vi "DAQ_PS Configure and Measure.vi"(0 "DAQmx Task In":refnum<k21>, 2 "Execution Settings":T4, 5 "Channel Settings":T7={"Voltage Setpoint(V)"=1.0, "Current Setpoint(A)"=0.1, "Remote Sense"=16095, "Idle Output Behavior"=15503, "Enable Output?"=TRUE} {"Idle Output Behavior" items=["Disable output when Task stopped"=15503, "Maintain Existing Value"=12528]; "Remote Sense" items=["Local"=16095, "Remote"=16096]; "Voltage Setpoint(V)" format="%.2p"; "Current Setpoint(A)" format="%.2p"}, 7 "Timing and Trigger Settings":T1={"Timing Settings"={"Sample Clock Source"="OnboardClock", "Sample Rate (Hz)"=10000.0, "Number of Samples"=1000, "Sample Timing Engine"=enum."Auto"}, "Trigger Settings"={"Trigger Select"=enum."No Trigger", "Digital Start Trigger Source"="", "Digital Start Trigger Edge"=10280}} {"Timing Settings"."Sample Rate (Hz)" format="%.2p"; "Trigger Settings"."Digital Start Trigger Edge" items=["Rising"=10280, "Falling"=10171]}, 11 "error in":errorcluster) -> (4 "DAQmx Task Out":refnum<k21>, 6 "Voltage Waveforms":waveform(dbl)(graph), 8 "Current Waveforms":waveform(dbl)(graph), 10 "Power Measurements":T6 {"Average Power (W)" format="%.2p"; "Max Power(W)" format="%.2p"; "Max Current Level(A)" format="%.2p"; "Max Voltage Level(V)" format="%.2p"}, 14 "Acquisition Time (s)":dbl format="%.2p", 15 "error out":errorcluster)   [LabVIEW 2021, in "DAQ_Power Supply Source and Measure.lvlib"]
doc: "Configures, Initiate and fetch results for power supply measurements"
uses:
  DAQ_Power Supply Source and Measure.lvlib
  Typedefs/Channel Settings.ctl
  Typedefs/Power Measurements.ctl
  Typedefs/Timing and Trigger Settings.ctl
  Typedefs/Timing Settings.ctl
  Typedefs/Trigger Settings.ctl
  Typedefs/Execution Settings.ctl
  Common/Typedefs/Execution Options - Measure.ctl
  <vilib>/DAQmx/read.llb/DAQmx Read (Power Wfm 1Chan NSamp).vi
  <vilib>/DAQmx/configure/timing.llb/DAQmx Timing (Sample Clock).vi
  <vilib>/DAQmx/configure/trigger.llb/DAQmx Start Trigger (Digital Edge).vi
  <vilib>/DAQmx/miscellaneous.llb/DAQmx Fill In Error Info.vi
  <resource>/objmgr/daqmx.rc
panel:
  # "Inputs"
  # "Outputs"
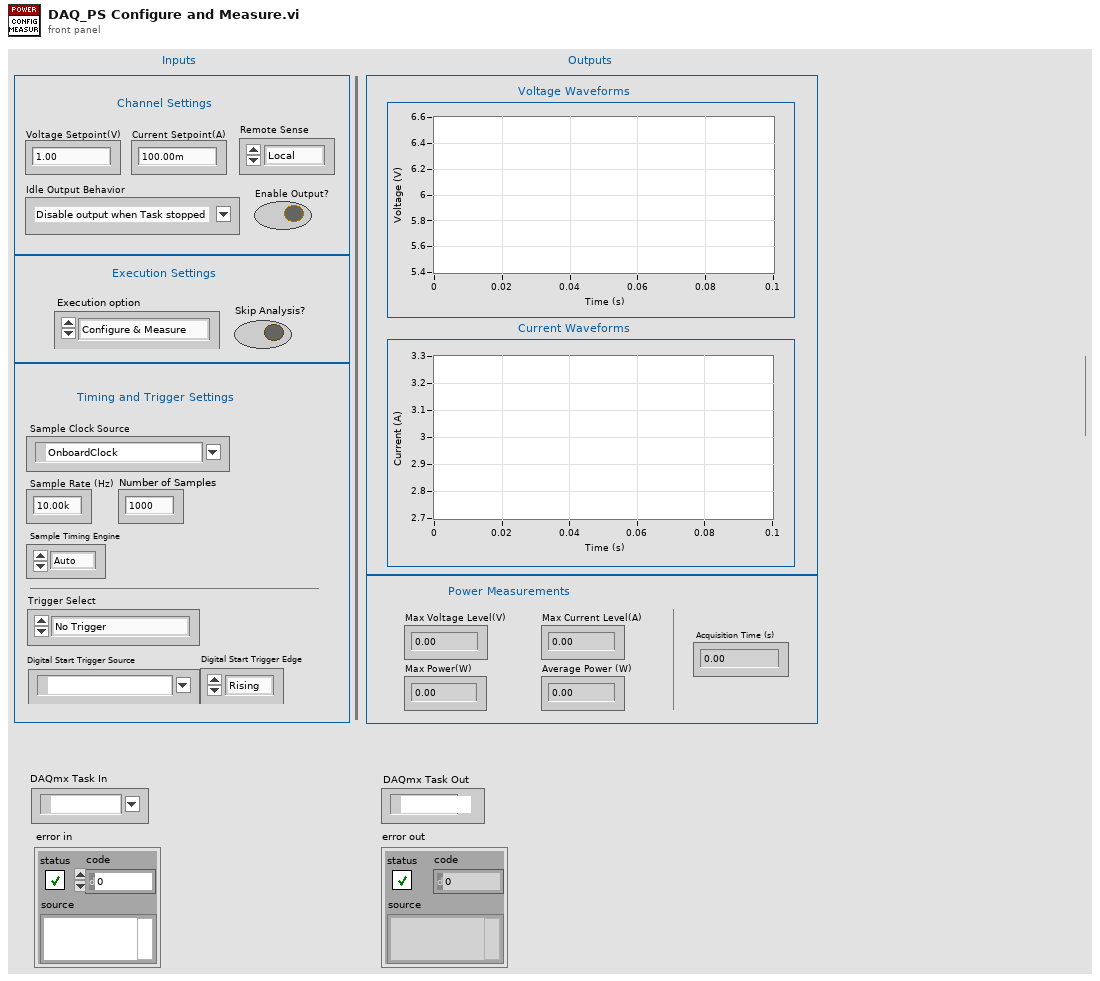
[diagram p1: front panel]
types:
  T1 = typedef "DAQ_Power Supply Source and Measure.lvlib/Timing and Trigger Settings.ctl" = cluster{"Timing Settings":T2, "Trigger Settings":T3}
  T2 = typedef "DAQ_Power Supply Source and Measure.lvlib/Timing Settings.ctl" = cluster{"Sample Clock Source":tag, "Sample Rate (Hz)":dbl, "Number of Samples":i32, "Sample Timing Engine":enum16{"te0", "te1", "ai", "Auto"}}
  T3 = typedef "DAQ_Power Supply Source and Measure.lvlib/Trigger Settings.ctl" = cluster{"Trigger Select":enum16{"No Trigger", "Digital Start"}, "Digital Start Trigger Source":tag, "Digital Start Trigger Edge":i32}
  T4 = typedef "DAQ_Power Supply Source and Measure.lvlib/Execution Settings.ctl" = cluster{"Execution option":T5, "Skip Analysis?":bool}
  T5 = typedef "Execution Options - Measure.ctl" = enum16{"Configure & Measure", "Configure only", "Measure only"}
  T6 = typedef "DAQ_Power Supply Source and Measure.lvlib/Power Measurements.ctl" = cluster{"Max Voltage Level(V)":dbl, "Max Current Level(A)":dbl, "Max Power(W)":dbl, "Average Power (W)":dbl}
  T7 = typedef "DAQ_Power Supply Source and Measure.lvlib/Channel Settings.ctl" = cluster{"Voltage Setpoint(V)":dbl, "Current Setpoint(A)":dbl, "Remote Sense":i32, "Idle Output Behavior":i32, "Enable Output?":bool}
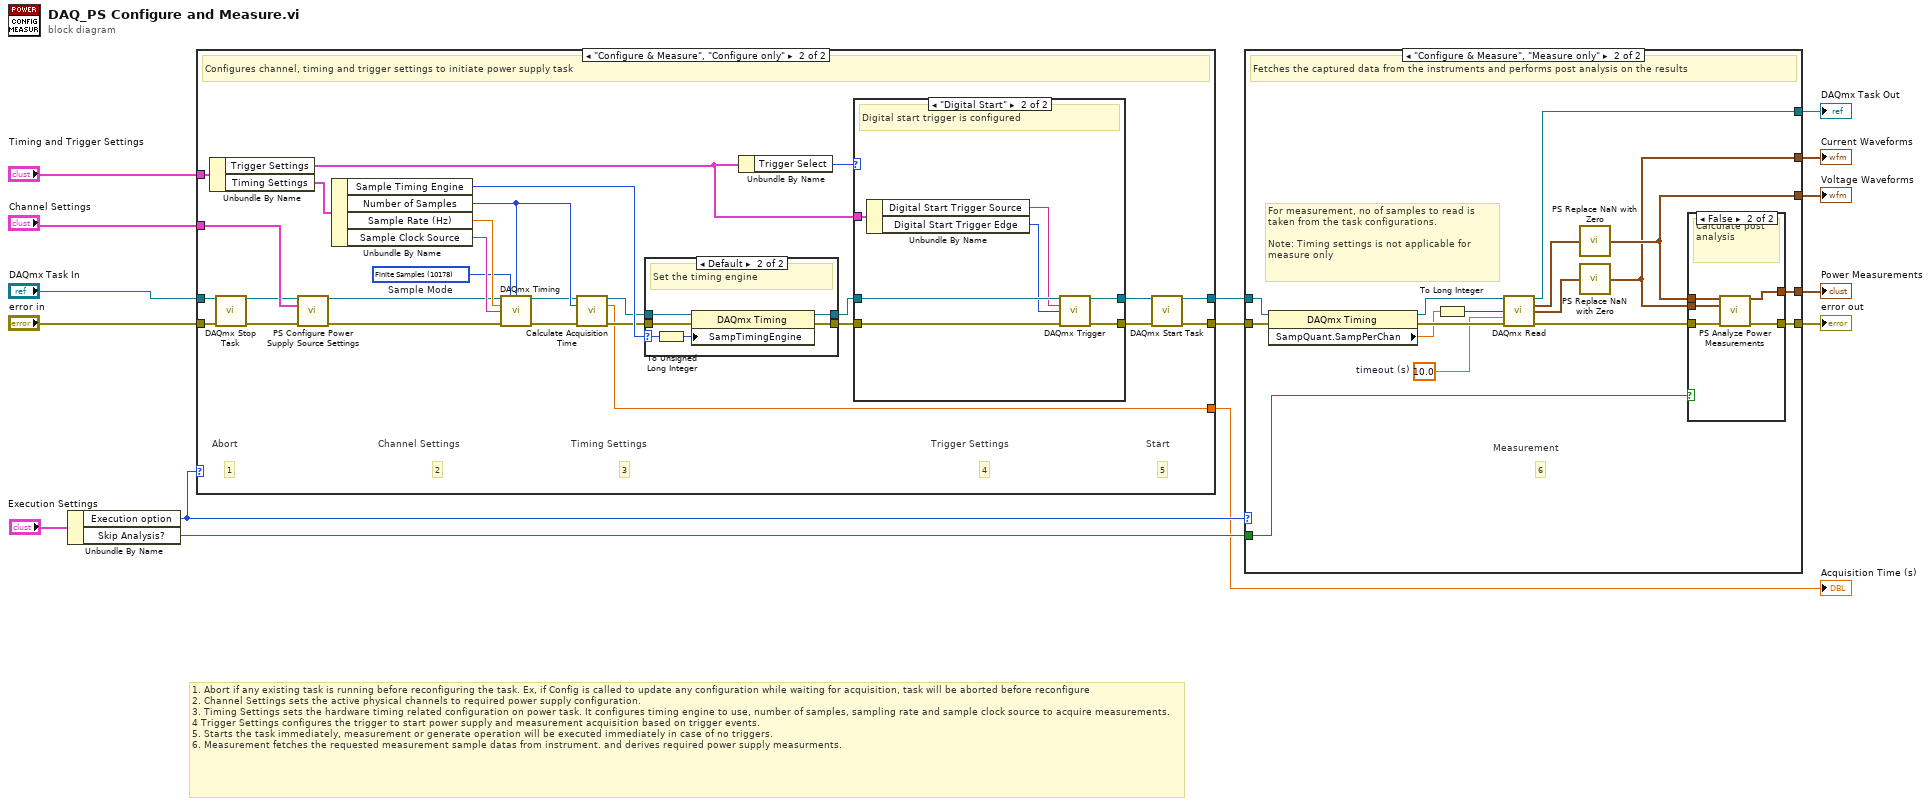
[diagram p0: block diagram]
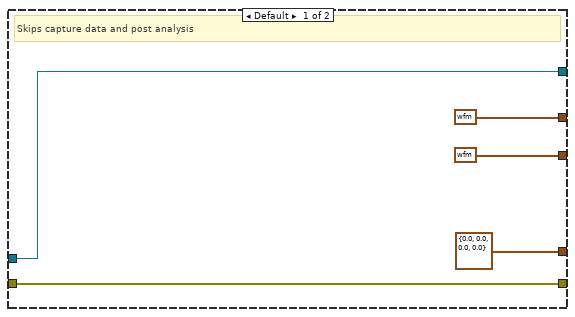
[diagram p5: hidden frame]
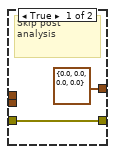
[diagram p6: hidden frame]
diagram:
  # "1. Abort if any existing task is running before reconfiguring the task. Ex, if Config is called to update any configuration while waiting for acquisition, task will be aborted before reconfigure\n2. Channel Settings sets the active physical channels to required power supply configuration.\n3. Timing Settings sets the hardware timing related configuration on power task. It configures timing engine to use, number of samples, sampling rate and sample clock source to acquire measurements.\n4 Trigger Settings configures the trigger to start power supply and measurement acquisition based on trigger events.\n5. Starts the task immediately, measurement or generate operation will be executed immediately in case of no triggers.\n6. Measurement fetches the requested measurement sample datas from instrument. and derives required power supply measurments."
  n1 = Unbundle By Name("Execution Settings") -> ("Execution option"=w5:T5, "Skip Analysis?"=w4:bool)
  n2 = case shown="\"Configure & Measure\", \"Configure only\"" w5 {
    tunnel: "Channel Settings" -> [_ w43]
    tunnel: "DAQmx Task In" -> [w16 w41]
    tunnel: "error in" -> [w17 w44]
    tunnel: [w16 w38] -> w10
    tunnel: [w17 w39] -> w9
    tunnel: "Timing and Trigger Settings" -> [_ w27]
    tunnel: [_ w18] -> w3
    frame Default {
      # "Configuration is skipped"
    }
    frame "Configure & Measure", "Configure only" {
      w29 = 10178 items=["Finite Samples"=10178, "Continuous Samples"=10123, "Hardware Timed Single Point"=12522]  # Sample Mode
      # "5"
      # "Start"
      # "1"
      # "Abort"
      # "4"
      # "Timing Settings"
      # "3"
      # "2"
      # "Trigger Settings"
      # "Channel Settings"
      # "Configures channel, timing and trigger settings to initiate power supply task"
      n3 = Unbundle By Name(w27) -> ("Trigger Settings"=w37:T3, "Timing Settings"=w35:T2)
      n4 = call <vilib>:"DAQmx Stop Task.vi"("task/channels in"=w41, "error in"=w44) -> ("task out"=w40:refnum<k21>, "error out"=w42:errorcluster)  [unwired: 12 in]
      n5 = call "PS Configure Power Supply Source Settings.vi"("DAQmx Task In"=w40, "Channel Settings"=w43, "error in (no error)"=w42) -> ("DAQmx Task Out"=w26:refnum<k21>, "error out"=w25:errorcluster)  [unwired: 11 in]
      n6 = Unbundle By Name(w35) -> ("Sample Timing Engine"=w34:enum16{"te0", "te1", "ai", "Auto"}, "Number of Samples"=w28:i32, "Sample Rate (Hz)"=w30:dbl, "Sample Clock Source"=w31:tag)
      n7 = call-poly <vilib>:"DAQmx Timing.vi"("task/channels in"=w26, "sample mode"=w29, "samples per channel"=w28, "rate"=w30, "source"=w31, "error in"=w25) -> ("task out"=w23:refnum<k21>, "error out"=w24:errorcluster)  [unwired: 8 in]
      n8 = call "Calculate Acquisition Time.vi"("Refnum in"=w23, "Number of Samples"=w28, "error in (no error)"=w24) -> ("Refnum out"=w21:refnum<k21>, "Acquisition Time Period (s)"=w18:dbl, "error out"=w22:errorcluster)  [unwired: 10 in]
      n9 = case shown="Default" w34 {
        selector: w34 -> [_ w50]
        tunnel: w22 -> [w46 w52]
        tunnel: w21 -> [w45 w51]
        tunnel: [w45 w49] -> w32
        tunnel: [w46 w48] -> w33
        frame "Auto" {
          # "Timing engine is auto-selected"
        }
        frame Default {
          # "Set the timing engine"
          n10 = To Unsigned Long Integer(number=w50) -> (unsigned 32bit integer=w47:u32)
          n11 = property class="DAQmx Timing"(reference=w51, error in=w52, "SampTimingEngine"=w47) -> (reference out=w49:refnum<k21>, error out=w48:errorcluster)
        }
      }
      n12 = Unbundle By Name(w37) -> ("Trigger Select"=w36:enum16{"No Trigger", "Digital Start"})
      n13 = case shown="\"Digital Start\"" w36 {
        tunnel: [w53 w61] -> w20
        tunnel: [w54 w60] -> w19
        tunnel: w33 -> [w53 w59]
        tunnel: w32 -> [w54 w58]
        tunnel: w37 -> [_ w57]
        frame Default {
          # "No Trigger settings has been configured"
        }
        frame "Digital Start" {
          # "Digital start trigger is configured"
          n14 = Unbundle By Name(w57) -> ("Digital Start Trigger Source"=w56:tag, "Digital Start Trigger Edge"=w55:i32)
          n15 = call-poly <vilib>:"DAQmx Trigger.vi"("task/channels in"=w58, "source"=w56, "edge"=w55, "error in"=w59) -> ("task out"=w60:refnum<k21>, "error out"=w61:errorcluster)  [unwired: 10 in]
        }
      }
      n16 = call <vilib>:"DAQmx Start Task.vi"("task/channels in"=w19, "error in"=w20) -> ("task out"=w38:refnum<k21>, "error out"=w39:errorcluster)  [unwired: 12 in]
    }
  }
  "Acquisition Time (s)" <- w3
  n17 = case shown="\"Configure & Measure\", \"Measure only\"" w5 {
    tunnel: w10 -> [w66 w78]
    tunnel: w9 -> [w65 w79]
    tunnel: [w66 w82] -> w14
    tunnel: [w65 w80] -> w11
    tunnel: [T6 {"Max Voltage Level(V)"=0.0, "Max Current Level(A)"=0.0, "Max Power(W)"=0.0, "Average Power (W)"=0.0} ("Power Measurements") w73] -> w7
    tunnel: w4 -> [_ w72]
    tunnel: [waveform(dbl) {"t0"=timestamp(0 s since 1904-01-01), "dt"=1.0, "Y"=[]} ("current") w68] -> w2
    tunnel: [waveform(dbl) {"t0"=timestamp(0 s since 1904-01-01), "dt"=1.0, "Y"=[]} ("voltage") w69] -> w1
    frame Default {
      # "Skips capture data and post analysis"
    }
    frame "Configure & Measure", "Measure only" {
      w67 = 10.0  # timeout (s)
      # "For measurement, no of samples to read is taken from the task configurations.\n\nNote: Timing settings is not applicable for measure only"
      # "6"
      # "Measurement"
      # "Fetches the captured data from the instruments and performs post analysis on the results"
      n18 = property class="DAQmx Timing"(reference=w78, error in=w79) -> (reference out=w77:refnum<k21>, error out=w76:errorcluster, "SampQuant.SampPerChan"=w75:dbl)
      n19 = To Long Integer(number=w75) -> (32bit integer=w74:i32)
      n20 = call-poly <vilib>:"DAQmx Read.vi"("task/channels in"=w77, "number of samples per channel"=w74, "timeout"=w67, "error in"=w76) -> ("task out"=w82:refnum<k21>, "voltage"=w70:waveform(dbl), "current"=w71:waveform(dbl), "error out"=w81:errorcluster)  [unwired: 8 in]
      n21 = call "PS Replace NaN with Zero.vi"("Input waveform"=w70) -> ("Output waveform"=w69:waveform(dbl))  [unwired: 14 in]
      n22 = call "PS Replace NaN with Zero.vi"("Input waveform"=w71) -> ("Output waveform"=w68:waveform(dbl))  [unwired: 14 in]
      n23 = case shown="False" w72 {
        tunnel: w81 -> [w84 w89]
        tunnel: [w84 w88] -> w80
        tunnel: w68 -> [_ w87]
        tunnel: w69 -> [_ w86]
        tunnel: [T6 {"Max Voltage Level(V)"=0.0, "Max Current Level(A)"=0.0, "Max Power(W)"=0.0, "Average Power (W)"=0.0} ("Power Measurements") w85] -> w73
        frame True {
          # "Skip post analysis"
        }
        frame False {
          # "Calculate post analysis"
          n24 = call "PS Analyze Power Measurements.vi"("Voltage Waveform In"=w86, "Current Waveform In"=w87, "error in (no error)"=w89) -> ("Power Measurements"=w85:T6, "error out"=w88:errorcluster)  [unwired: 11 in]
        }
      }
    }
  }
  "DAQmx Task Out" <- w14
  "error out" <- w11
  "Power Measurements" <- w7
  "Voltage Waveforms" <- w1
  "Current Waveforms" <- w2
